vi "Determine Vision Shot Setpoints.vi"(4 "Vision Aligned?":bool, 5 "x^2":dbl, 6 "Init?":bool, 7 "x":dbl, 8 "Current Angle":dbl, 10 "c":dbl, 11 "Distance from Target":dbl) -> (2 "Angle":dbl)   [LabVIEW 2015]
uses:
  Common Code/Change Detect Boolean.vi
  Robot Global Data.vi
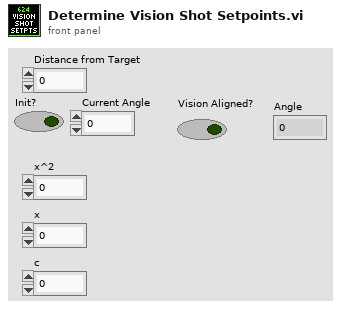
[diagram p1: front panel]
types:
  T1 = typedef "Drivetrain Status Cluster.ctl" = cluster{"Modes":T2, "Y (Throttle)":dbl, "X (Steer)":dbl, "Gyro In Range?":bool, "Distance Drive Finished?":bool, "Stop Eject Lockout":bool, "Dist Drive Status":T3, "Y Target":dbl, "Heading Target":dbl, "Vision Target Aligned?":bool, "Gear":dbl, "1st Gear Time":dbl, "2nd Gear Time":dbl, "1st Gear Shifts":dbl, "2nd Gear Shifts":dbl}
  T2 = typedef "Drivetrain Modes.ctl" = enum16{"Tank", "Climb", "Manual", "Goal Vision Targeting", "PID Distance Drive", "Hybrid", "Gyro Steer"}
  T3 = typedef "Dist Drive Status.ctl" = cluster{"Y In Range":bool, "X In Range":bool, "Gyro In Range":bool, "Y Dist":dbl, "X Dist":dbl, "Gyro":dbl}
  T4 = typedef "Dashboard Control Data.ctl" = cluster{"Shooter Presets":T5, "Encoder Control":T7, "Steer PID output":cluster{"output high":dbl, "output low":dbl}, " Steer PID gains":cluster{"proportional gain (Kc)":dbl, "integral time (Ti, min)":dbl, "derivative time (Td, min)":dbl}, "Drivetrain Settings":T8, "Vision Packet":T9, "Dashboard Drivetrain Command":T10, "Info/Command Cluster":T12, "Ball Vision Packet":T13, "Intake Presets":T15, "Intake Encoder Control":T17, "Climb Presets":T18, "Goal Output Range":cluster{"output high":dbl, "output low":dbl}, "Enabled Systems":T19, "Auton Presets":T20, "Pressure M":dbl, "Pressure B":dbl}
  T5 = typedef "Shooter Presets.ctl" = cluster{"Batter Shot":T6, "Deep Middle":T6, "Manual Shot":T6, "Left Ticks Per Rotation":dbl, "Right Ticks Per Rotation":dbl, "Low Bar Shot":T6, "Shooter RPM Tolerance":dbl, "IIR Filter Power":dbl, "Trigger Power":dbl, "Fire from Load Delay":i32, "Max Angle":dbl, "Min Angle":dbl, "Angle PID gains":cluster{"P":dbl, "I":dbl, "D":dbl}, "Angle Output":cluster{"output high":dbl, "output low":dbl}, "Shooter Angle Tolerance":dbl, "Vision Shoot x^2":dbl, "Vision Shoot x":dbl, "IR Let Go Timer":dbl, "High Goal Center Height":dbl, "Feed Forward Max Accel":dbl, "Feed Forward Kv":dbl, "Backwards Trigger":dbl, "Shot Finish Delay (ms)":dbl, "Angle Max Current":dbl, "Angle Current Trip Time":dbl, "Intake Angle":dbl, "Vision Shoot c":dbl, "Reset?":bool, "Servo Release Delay":dbl, "Servo Idle Angle":i32, "Servo Hold Angle":i32, "Angle Pot x":dbl, "Angle Pot c":dbl, "Ignore Angle?":bool, "Manual Output?":bool, "Manual Out":dbl, "Max RPM":dbl, "Safty Frist Angle":dbl, "Intake Danger Height":dbl, "Angle Pot B":i32, "Angle Pot M":dbl, "FF Finish RPM":dbl, "RPM PID Right":cluster{"P":dbl, "I":dbl, "D":dbl, "FF":dbl}, "RPM PID Left":cluster{"P":dbl, "I":dbl, "D":dbl, "FF":dbl}, "Backwards RPM":dbl, "Vision RPM":dbl, "Run Wheels Backward Delay":u32, "Cleat Shot":T6}
  T6 = typedef "Shot Presets.ctl" = cluster{"L":dbl, "R":dbl, "A":dbl}
  T7 = typedef "Encoder Control.ctl" = cluster{"Right Tick Constant":dbl, "Left Tick Constant":dbl, "Reset?":bool, "Y Dist":cluster{"PID gains":cluster{"proportional gain (Kc)":dbl, "integral time (Ti, min)":dbl, "derivative time (Td, min)":dbl}}, "Y Stop Thresh":dbl, "Y Stop Speed":dbl}
  T8 = typedef "Drivetrain Settings.ctl" = cluster{"Gyro Tolerance":dbl, "Throttle Ramp (ms)":dbl, "Angular rate compensation":bool, "Throttle to Rate Scale":dbl, "Rate compensation gain":dbl, "Kv":dbl, "Ka":dbl, "Feed Forward P":dbl, "Feed Forward D":dbl, "Goal Vision PID gains":cluster{"proportional gain (Kc)":dbl, "integral time (Ti, min)":dbl, "derivative time (Td, min)":dbl}, "Goal Detection Window":dbl, "Creep Rate":dbl, "Vision Throttle Threshold":dbl}
  T9 = typedef "Goal Vision Packet.ctl" = cluster{"Distance":dbl, "Center X":dbl, "Center Y":dbl, "Found Target?":bool, "Robot Center":dbl, "Angle":dbl}
  T10 = typedef "Dashboard Drivetrain Command.ctl" = cluster{"Drivetrain Vision":T11}
  T11 = typedef "Drivetrain Vision.ctl" = cluster{"Goal Window":dbl, "Ball Window":dbl}
  T12 = typedef "Ball Tracking Command Cluster.ctl" = cluster{"Distance to Ball":dbl, "Desired Angle":dbl, "Command":enum16{"Turn to Ball", "Turn to Angle", "Get Distance"}, "Pixels from Center":dbl}
  T13 = typedef "Ball Vision Packet.ctl" = cluster{"Ball Detected?":bool, "Distance to Ball":dbl, "Desired Angle":dbl, "Pixels from Center":dbl, "Tracking mode":T14}
  T14 = typedef "Tracking Mode.ctl" = enum16{"Turn to Ball", "Turn to Angle"}
  T15 = typedef "Intake Presets.ctl" = cluster{"Intake Speed":dbl, "Outake Speed":dbl, "Low Height":dbl, "Half Height":dbl, "Full Height":dbl, "Angle Speed":dbl, "Angle Tolerance":dbl, "Encoder Scale":dbl, "Load Height":dbl, "Output Range":T16, "Rotation Power Max/Min":dbl, "MaxCurrent":dbl, "Intake Trip Time":dbl, "Idle Height":dbl, "Max Height":dbl, "Reset Encoders?":bool, "PID gains":cluster{"proportional gain (Kc)":dbl, "integral time (Ti, min)":dbl, "derivative time (Td, min)":dbl}, "Intake Stop Delay":u32}
  T16 = typedef "Drivetrain Output Range.ctl" = cluster{"output high":dbl, "output low":dbl}
  T17 = typedef "IntakeEcoderControl.ctl" = cluster{"Arm Tick Constant":dbl, "Reset?":bool, "Y Dist":cluster{"PID gains":cluster{"proportional gain (Kc)":dbl, "integral time (Ti, min)":dbl, "derivative time (Td, min)":dbl}}, "Y Stop Thresh":dbl, "Y Stop Speed":dbl}
  T18 = typedef "Climb Presets.ctl" = cluster{"Pull Power":dbl, "Time to Hold":dbl, "Extend Power":dbl}
  T19 = typedef "Enabled Systems.ctl" = cluster{"Shoot":bool, "Intake":bool, "DT":bool, "Gyro":bool, "100ms":bool, "US":bool}
  T20 = typedef "Autonomous Presets.ctl" = cluster{"Pitch Limit":dbl, "Roll Limit":dbl, "Ultrasonic Limit":dbl, "Start Position":dbl, "Cross Position":dbl}
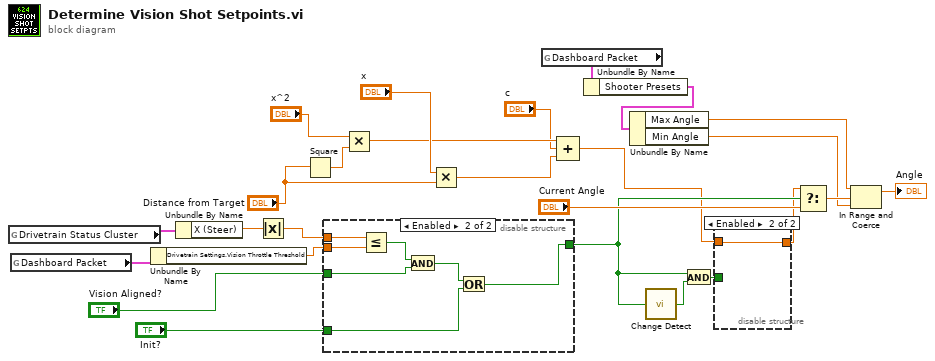
[diagram p0: block diagram]
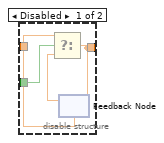
[diagram p2: hidden frame]
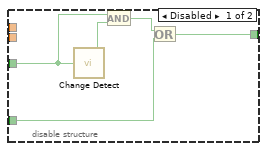
[diagram p3: hidden frame]
diagram:
  n1 = global read "Robot Global Data.vi" "Drivetrain Status Cluster"() -> (w16:T1)
  n2 = global read "Robot Global Data.vi" "Dashboard Packet"() -> (w15:T4)
  n3 = Unbundle By Name(w15) -> ("Drivetrain Settings.Vision Throttle Threshold"=w14:dbl)
  n4 = Unbundle By Name(w16) -> ("X (Steer)"=w17:dbl)
  n5 = Absolute Value(x=w17) -> (abs(x)=w6:dbl)
  n6 = Square(x="Distance from Target") -> (x^2=w26:dbl)
  n7 = disable-structure shown="Enabled" {
    disable-tunnel: "Vision Aligned?" -> [w30 w38]
    disable-tunnel: "Init?" -> [w28 w33]
    disable-tunnel: [w27 w32] -> w3
    disable-tunnel: w6 -> [_ w37]
    disable-tunnel: w14 -> [_ w36]
    frame Disabled {
      n8 = call-poly "Change Detect.vi"("In"=w30) -> ("Changed?"=w31:bool)
      n9 = And(x=w30, y=w31) -> (x .and. y?=w29:bool)
      n10 = Or(x=w29, y=w28) -> (x .or. y?=w27:bool)
    }
    frame Enabled {
      n11 = Less Or Equal?(x=w37, y=w36) -> (x <= y?=w35:bool)
      n12 = And(x=w35, y=w38) -> (x .and. y?=w34:bool)
      n13 = Or(x=w34, y=w33) -> (x .or. y?=w32:bool)
    }
  }
  n14 = Multiply(x="x^2", y=w26) -> (x*y=w22:dbl)
  n15 = Multiply(x="x", y="Distance from Target") -> (x*y=w20:dbl)
  n16 = global read "Robot Global Data.vi" "Dashboard Packet"() -> (w10:T4)
  n17 = Compound Arithmetic op=ADD(w22, "c", w20) -> (w1:dbl)
  n18 = Unbundle By Name(w10) -> ("Shooter Presets"=w9:T5)
  n19 = Unbundle By Name(w9) -> ("Max Angle"=w8:dbl, "Min Angle"=w7:dbl)
  n20 = call-poly "Change Detect.vi"("In"=w3) -> ("Changed?"=w5:bool)
  n21 = And(x=w3, y=w5) -> (x .and. y?=w4:bool)
  n22 = disable-structure shown="Enabled" {
    disable-tunnel: w4 -> [w42 _]
    disable-tunnel: [w40 w43] -> w2
    disable-tunnel: w1 -> [w39 w43]
    frame Disabled {
      n23 = feedback #1(w39) -> (w41:dbl)
      n24 = Select(t=w39, s=w42, f=w41) -> (s? t:f=w40:dbl)
      n25 = feedback-in #1(w40) -> ()
    }
    frame Enabled {
    }
  }
  n26 = Select(t=w2, s=w3, f="Current Angle") -> (s? t:f=w12:dbl)
  n27 = In Range and Coerce(upper limit=w8, x=w12, lower limit=w7) -> (coerced(x)=→"Angle":dbl)  [unwired: 1 out]
